vi "Double Mean.vi"(11 "Double Array":dbl[](array[numeric])) -> (3 "Numeric":dbl)   [LabVIEW 2014]
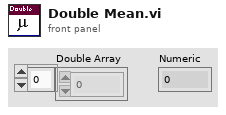
[diagram p1: front panel]
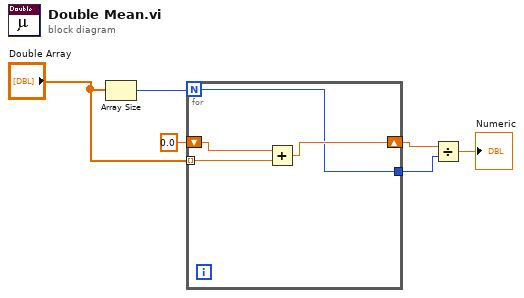
[diagram p0: block diagram]
diagram:
  n1 = Array Size(array="Double Array") -> (size(s)=w2:i32)
  n2 = for {
    N: w2 -> [w7]
    shift-right: [w8] -> w3
    shift-left: 0.0 -> [w10]
    tunnel: "Double Array" -> [w9] mode=indexing
    tunnel: [w7] -> w4
    n3 = Add(x=w10, y=w9) -> (x+y=w8:dbl)
  }
  n4 = Divide(x=w3, y=w4) -> (x/y=→"Numeric":dbl)
